vi "BruteForceSynthesis.vi"() -> (2 "timed out?":bool, 3 "Key Position \non a 102 key \nPiano":u8)   [LabVIEW 2016]
uses:
  <vilib>/sound2/lvsound2.llb/Sound Data Format.ctl
  <vilib>/sound2/lvsound2.llb/Sampling Mode.ctl
  <vilib>/express/express analysis/Spectral/Block/exnSpectralBlock spectral measurements power poly.vi
  <vilib>/express/express analysis/Spectral/Block/exnSpectralBlock spectral measurements power WFM.vi
  <vilib>/sound2/lvsound2.llb/Sound Output Set Volume (Single).vi
  <vilib>/sound2/lvsound2.llb/Sound Output Write (DBL).vi
  <vilib>/express/express analysis/Spectral/XNode/ExpressSpectralMeasurementsBlockNode.xnode
panel:
  in  "Volume":dbl(slide)=28.782816229116946 scale=20.0..100.0
  out "Power Spectrum":cluster{"f0":dbl, "df":dbl, "magnitude":dbl[]}(graph)
  in  "?":bool
  in  "Third Harmonic":T1(ring)
  in  "Second Harmonic":T1(ring)=enum."Triangle Wave"
  in  "Fundamental":T1(ring)=enum."Sawtooth Wave"
  in  "A third":T1(ring)=enum."Square Wave"
  in  "A second":T1(ring)
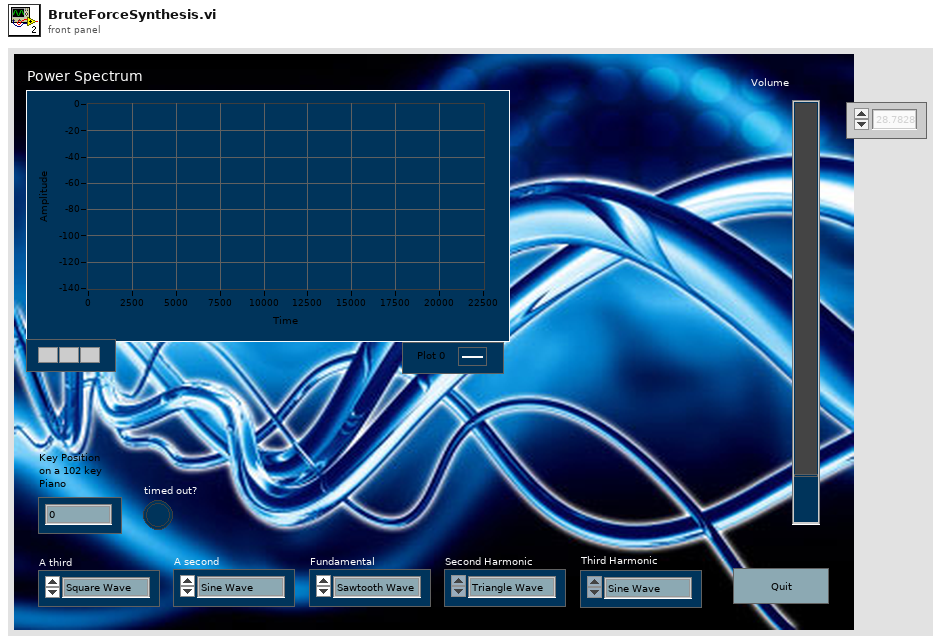
[diagram p1: front panel]
types:
  T1 = enum16{"Sine Wave", "Triangle Wave", "Square Wave", "Sawtooth Wave"}
  T2 = typedef "Sound Data Format.ctl" = cluster{"sample rate (S/s)":dbl, "number of channels":i32, "bits per sample":i32}
  T3 = cluster{"averaging mode":u16, "weighting mode":u16, "number of averages":u32}
  T4 = cluster{"dB On (F)":bool, "unwrap phase (F)":bool, "convert to degree (F)":bool}
  T5 = typedef "Sampling Mode.ctl" = i32
  T6 = typedef "Sound Output Task ID.ctl" = u32
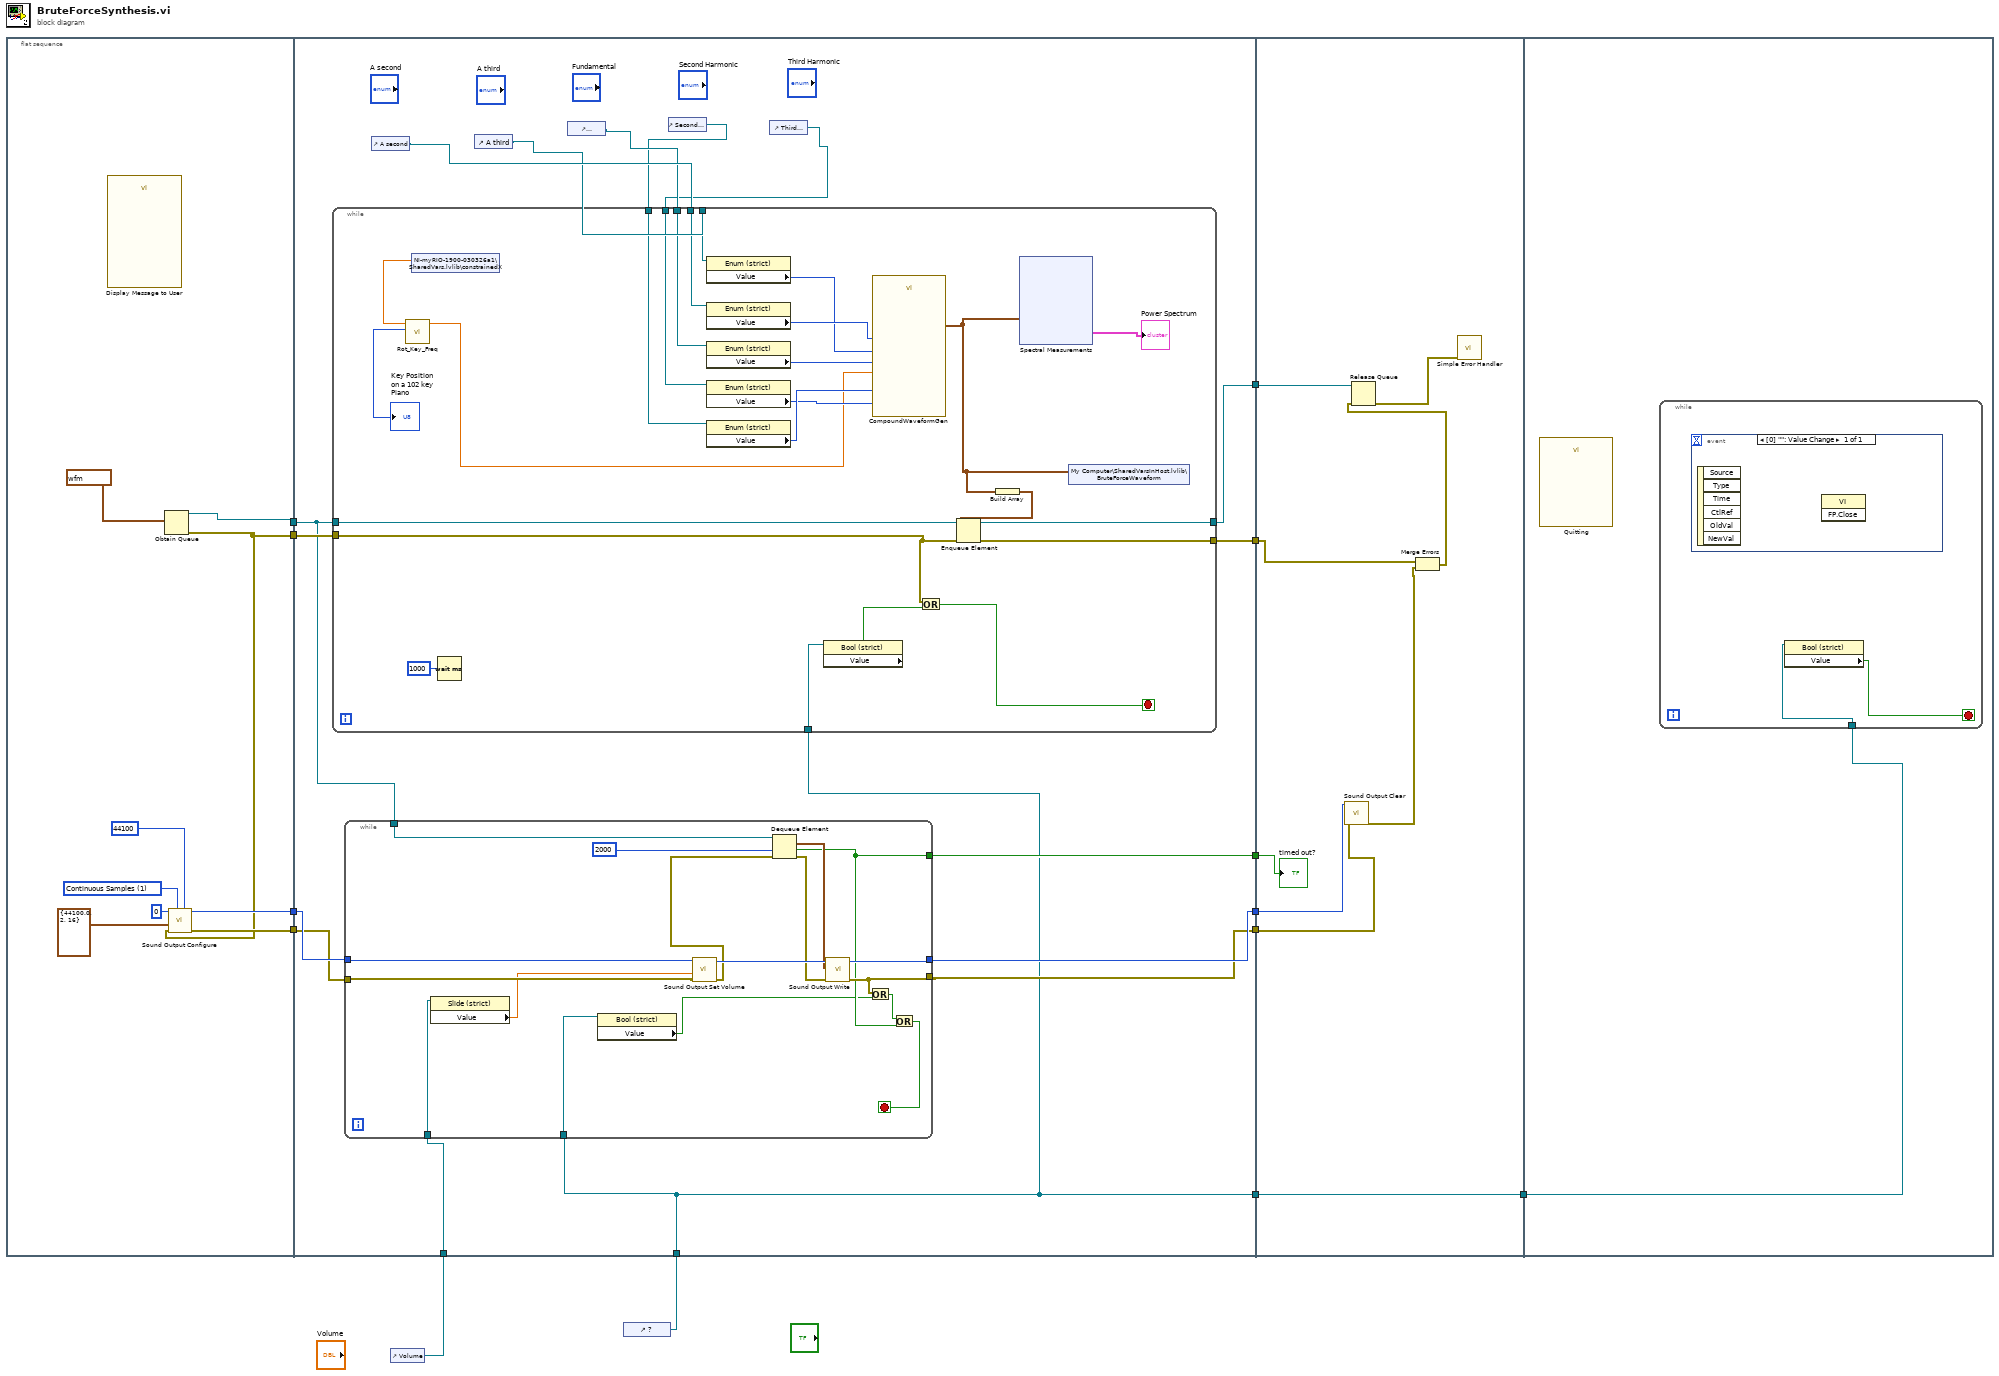
[diagram p0: block diagram]
diagram:
  n1 = flat-sequence {
    tunnel: [w19] -> w13
    tunnel: [w18] -> w12
    tunnel: [w15] -> w9
    tunnel: [w14] -> w8
    tunnel: w13 -> [w38]
    tunnel: w12 -> [w37]
    tunnel: [w36] -> w11
    tunnel: [w35] -> w10
    tunnel: w9 -> [w33]
    tunnel: w8 -> [w34]
    tunnel: [w32] -> w7
    tunnel: [w31] -> w6
    tunnel: [w30] -> w5
    tunnel: w1 -> [w24]
    tunnel: w4 -> [w23]
    tunnel: [w23] -> w2
    tunnel: w11 -> [w94]
    tunnel: w10 -> [w93]
    tunnel: w7 -> [w92]
    tunnel: w6 -> [w91]
    tunnel: w5 -> [w90]
    tunnel: [w89] -> w3
    tunnel: w2 -> [w89]
    tunnel: w3 -> [w98]
    frame #0 {
      w22 = T5 1 items=["Finite Samples", "Continuous Samples"] ("sample mode")
      n2 = call "Display Message to User"() -> ()  [unwired: 10 in, 2 out]
      n3 = Obtain Queue(element data type=waveform(dbl)[] [{"t0"=timestamp(3482746353.0334034 s since 1904-01-01), "dt"=4.5351473922902495e-05, "Y"=array[5000 elements]}, {"t0"=timestamp(3482746353.0334034 s since 1904-01-01), "dt"=4.5351473922902495e-05, "Y"=array[5000 elements]}] ("Generated Sound")) -> (queue out=w15:refnum<queue>, error out=w14:errorcluster)  [unwired: 4 in, 1 out]
      n4 = call <vilib>:"Sound Output Configure.vi"("number of samples/ch"=44100, "sample mode"=w22, "error in (no error)"=w14, "sound format"=T2 {"sample rate (S/s)"=44100.0, "number of channels"=2, "bits per sample"=16}, "device ID"=u32 0) -> ("error out"=w18:errorcluster, "task ID"=w19:T6)  [unwired: 5 in]
    }
    frame #1 {
      n5 = while {
        tunnel: w38 -> [w54]
        tunnel: w37 -> [w53]
        tunnel: w24 -> [w52]
        tunnel: w23 -> [w51]
        tunnel: [w50] -> w36
        tunnel: [w49] -> w35
        tunnel: w33 -> [w44]
        tunnel: [w41] -> w32
        stop <- w42 stop-if-true
        n6 = property class="Slide (strict)"(reference=w52) -> ("Value"=w39:dbl)  [unwired: 1 in, 2 out]
        n7 = property class="Bool (strict)"(reference=w51) -> ("Value"=w40:bool)  [unwired: 1 in, 2 out]
        n8 = call-poly <vilib>:"Sound Output Set Volume.vi"("error in (no error)"=w53, "volume"=w39, "task ID"=w54) -> ("error out"=w46:errorcluster, "task ID out"=w55:T6)  [unwired: 7 in]
        n9 = Dequeue Element(queue=w44, timeout in ms (-1)=2000, error in (no error)=w46) -> (element=w43:waveform(dbl)[], timed out?=w41:bool, error out=w45:errorcluster)  [unwired: 1 out]
        n10 = call-poly <vilib>:"Sound Output Write.vi"("error in (no error)"=w45, "data"=w43, "task ID"=w55) -> ("error out"=w49:errorcluster, "task ID out"=w50:T6)  [unwired: 7 in]
        n11 = Or(x=w49, y=w40) -> (x .or. y?=w48:bool)
        n12 = Or(x=w48, y=w41) -> (x .or. y?=w42:bool)
      }
      n13 = control-ref of="A second"() -> (w29:refnum<vi>)
      n14 = control-ref of="A third"() -> (w28:refnum<vi>)
      n15 = control-ref of="Fundamental"() -> (w27:refnum<vi>)
      n16 = control-ref of="Second Harmonic"() -> (w26:refnum<vi>)
      n17 = control-ref of="Third Harmonic"() -> (w25:refnum<vi>)
      n18 = while {
        tunnel: w28 -> [w77]
        tunnel: w29 -> [w76]
        tunnel: w27 -> [w75]
        tunnel: w25 -> [w74]
        tunnel: w26 -> [w73]
        tunnel: w33 -> [w67]
        tunnel: w34 -> [w66]
        tunnel: [w65] -> w31
        tunnel: [w64] -> w30
        tunnel: w23 -> [w62]
        stop <- w68 stop-if-true
        n19 = shared-variable "NI-myRIO-1900-030326a1\\SharedVars.lvlib\\constrainedX"() -> (w79:dbl)  [unwired: 1 in, 1 out]
        n20 = call "Rot_Key_Freq.vi"("Rotation"=w79) -> ("Key Position"=→"Key Position \non a 102 key \nPiano":u8, "Fundamental Frequency"=w61:dbl)  [unwired: 9 in]
        n21 = Wait (ms)(milliseconds to wait=u32 1000) -> ()  [unwired: 1 out]
        n22 = property class="Enum (strict)"(reference=w77) -> ("Value"=w58:T1)  [unwired: 1 in, 2 out]
        n23 = property class="Enum (strict)"(reference=w76) -> ("Value"=w59:T1)  [unwired: 1 in, 2 out]
        n24 = property class="Enum (strict)"(reference=w75) -> ("Value"=w72:T1)  [unwired: 1 in, 2 out]
        n25 = property class="Enum (strict)"(reference=w74) -> ("Value"=w70:T1)  [unwired: 1 in, 2 out]
        n26 = property class="Enum (strict)"(reference=w73) -> ("Value"=w71:T1)  [unwired: 1 in, 2 out]
        n27 = property class="Bool (strict)"(reference=w62) -> ("Value"=w69:bool)  [unwired: 1 in, 2 out]
        n28 = call "CompoundWaveformGen.vi"("Fundamental Frequency"=w61, "Third Harmonic"=w70, "A third"=w58, "A second"=w59, "Fundamental"=w72, "Second Harmonic"=w71) -> ("signal out"=w57:waveform(dbl))  [unwired: 9 in]
        n29 = Or(x=w66, y=w69) -> (x .or. y?=w68:bool)
        n30 = Build Array(w57) -> (w63:waveform(dbl)[])
        n31 = Enqueue Element(queue=w67, element=w63, error in (no error)=w66) -> (queue out=w64:refnum<queue>, error out=w65:errorcluster)  [unwired: 1 in, 1 out]
        n32 = xnode "Spectral Measurements"("Signals"=w57) -> ("Power Spectrum"=→"Power Spectrum":cluster{"f0":dbl, "df":dbl, "magnitude":dbl[]})  [unwired: 1 in, 1 out]
        n33 = shared-variable "My Computer\\SharedVarsInHost.lvlib\\BruteForceWaveform"(w57) -> ()  [unwired: 1 in, 1 out]
      }
    }
    frame #2 {
      n34 = call <vilib>:"Sound Output Clear.vi"("error in (no error)"=w93, "task ID"=w94) -> ("error out"=w95:errorcluster)  [unwired: 9 in]
      n35 = Merge Errors(w91, w95) -> (w97:errorcluster)
      n36 = Release Queue(queue=w90, error in (no error)=w97) -> (error out=w96:errorcluster)  [unwired: 1 in, 2 out]
      n37 = call <vilib>:"Simple Error Handler.vi"("error in (no error)"=w96) -> ()  [unwired: 4 in, 5 out]
      "timed out?" <- w92
    }
    frame #3 {
      n38 = call "Quitting"() -> ()  [unwired: 10 in, 2 out]
      n39 = while {
        tunnel: w98 -> [w100]
        stop <- w99 stop-if-true
        n40 = event shown="[0] \"\": Value Change" {
          selector: _ -> [_]
          dyn-events: _ -> [_]
          timeout: _ -> [_]
          event Value Change {
            n41 = event-data() -> ()  [unwired: 1 in, 6 out]
            n42 = invoke class="VI" method="FP.Close"() -> ()  [unwired: 3 in, 3 out]
          }
        }
        n43 = property class="Bool (strict)"(reference=w100) -> ("Value"=w99:bool)  [unwired: 1 in, 2 out]
      }
    }
  }
  n44 = control-ref of="Volume"() -> (w1:refnum<vi>)
  n45 = control-ref of="?"() -> (w4:refnum<vi>)
